vi "Stop Core.vi"(10 "final error code":i32, 11 "Chronometer in":refnum<class "Chronometer.lvclass">) -> (3 "Chronometer out":refnum<class "Chronometer.lvclass">)   [LabVIEW 2023, in "Chronometer.lvlib" / "Chronometer.lvclass"]
uses:
  Chronometer.lvclass
  builds/Tools/Config.lvlibp/Config.lvclass
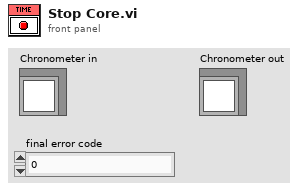
[diagram p1: front panel]
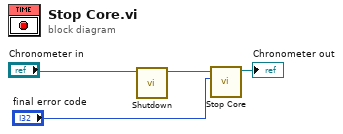
[diagram p0: block diagram]
diagram:
  n1 = call "Shutdown.vi"("Chronometer in"="Chronometer in") -> ("Chronometer out"=w1:refnum<class "Chronometer.lvclass">)  [unwired: 9 in, 1 out]
  n2 = call-parent "Stop Core.vi"("final error code"="final error code", "Monitored Actor in"=w1) -> ("Monitored Actor out"=→"Chronometer out":refnum<class "Chronometer.lvclass">)  [unwired: 9 in]
